vi "GetType.vi"(8 "error in (no error)":errorcluster, 11 "Configure FM Internal [FM] Msg in":refnum<class "Configure FM Internal [FM] Msg.lvclass">) -> (0 "error out":errorcluster, 2 "Data Sample":variant, 3 "Configure FM Internal [FM] Msg out":refnum<class "Configure FM Internal [FM] Msg.lvclass">)   [LabVIEW 2014, in "CS++Fgen.lvlib" / "Configure FM Internal [FM] Msg.lvclass"]
doc: "This VI delivers a sample of the data type format the message expects."
uses:
  Configure FM Internal [FM] Msg.lvclass
  Configure FM Internal [FM] Msg.lvclass/Configure FM Internal [FM] Msg.ctl
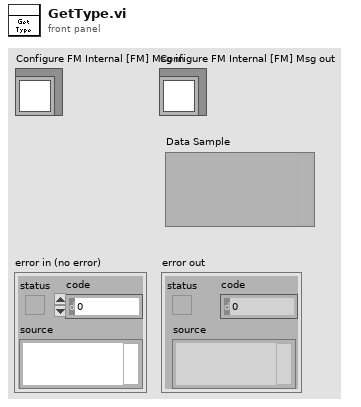
[diagram p1: front panel]
types:
  T1 = cluster{"modulation waveform (Sine)":i32, "peak deviation (100 Hz)":dbl[unit], "modulation frequency (1000 Hz)":dbl[unit]}
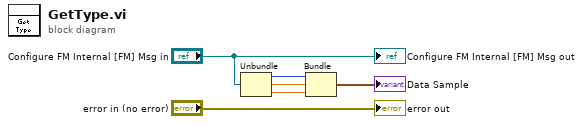
[diagram p0: block diagram]
diagram:
  n1 = Unbundle("Configure FM Internal [FM] Msg in") -> (w4:i32, w3:dbl[unit], w2:dbl[unit])
  n2 = Bundle("modulation waveform (Sine)"=w4, "peak deviation (100 Hz)"=w3, "modulation frequency (1000 Hz)"=w2) -> (→"Data Sample":T1)  [unwired: 1 in]
  "error out" <- "error in (no error)"
  "Configure FM Internal [FM] Msg out" <- "Configure FM Internal [FM] Msg in"
